vi "DAQmx.Dark.Current.SubVI.GenerateBooleanArray.vi"(8 "Activate: 1\nDeactivate: 0":bool, 11 "Tube":u8) -> (3 "Boolean array":bool[](array[boolean]))   [LabVIEW 2020]
panel:
  # "___"
  # "___"
  # "___"
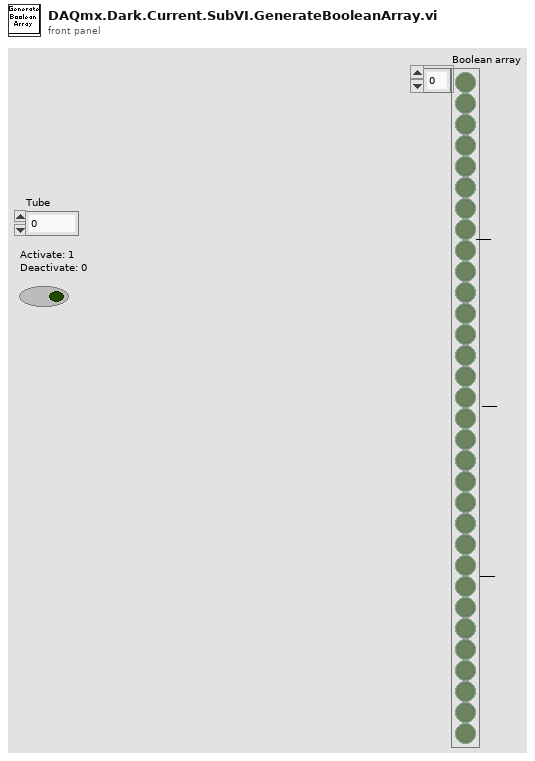
[diagram p1: front panel]
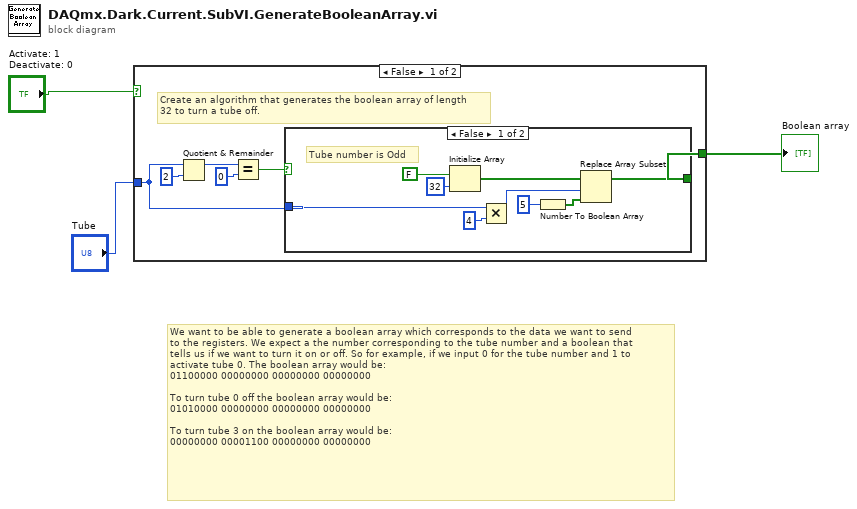
[diagram p0: block diagram]
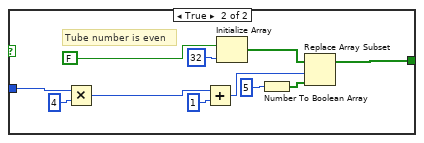
[diagram p2: hidden frame]
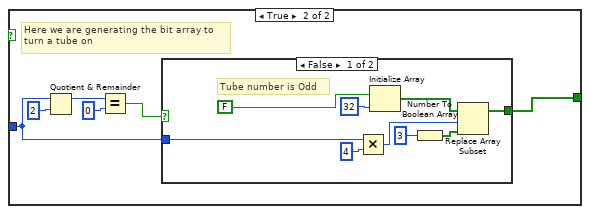
[diagram p3: hidden frame]
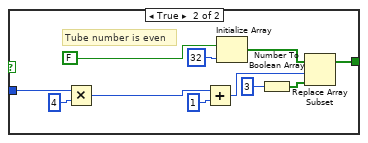
[diagram p4: hidden frame]
diagram:
  # "We want to be able to generate a boolean array which corresponds to the data we want to send \nto the registers. We expect a the number corresponding to the tube number and a boolean that\ntells us if we want to turn it on or off. So for example, if we input 0 for the tube number and 1 to\nactivate tube 0. The boolean array would be:\n01100000 00000000 00000000 00000000 \n\nTo turn tube 0 off the boolean array would be:\n01010000 00000000 00000000 00000000\n\nTo turn tube 3 on the boolean array would be:\n00000000 00001100 00000000 00000000"
  n1 = case shown="False" "Activate: 1\nDeactivate: 0" {
    tunnel: "Tube" -> [w5 w34]
    tunnel: [w6 w35] -> w1
    frame False {
      # "Create an algorithm that generates the boolean array of length\n32 to turn a tube off."
      n2 = Quotient & Remainder(x=w5, y=2) -> (x-y*floor(x/y)=w8:i32)  [unwired: 1 out]
      n3 = Equal?(x=w8, y=0) -> (x = y?=w4:bool)
      n4 = case shown="False" w4 {
        tunnel: w5 -> [w16 w24]
        tunnel: [w10 w25] -> w6
        frame False {
          # "Tube number is Odd"
          n5 = Initialize Array(FALSE, 32) -> (w12:bool[])
          n6 = Multiply(x=w16, y=4) -> (x*y=w11:i32)
          n7 = Number To Boolean Array(number=5) -> (Boolean array=w15:bool[])
          n8 = Replace Array Subset(array=w12, new element=w15, index=w11) -> (w10:bool[])
        }
        frame True {
          # "Tube number is even"
          n9 = Multiply(x=w24, y=4) -> (x*y=w20:i32)
          n10 = Add(x=w20, y=1) -> (x+y=w21:i32)
          n11 = Initialize Array(FALSE, 32) -> (w27:bool[])
          n12 = Number To Boolean Array(number=5) -> (Boolean array=w22:bool[])
          n13 = Replace Array Subset(array=w27, new element=w22, index=w21) -> (w25:bool[])
        }
      }
    }
    frame True {
      # "Here we are generating the bit array to \nturn a tube on"
      n14 = Quotient & Remainder(x=w34, y=2) -> (x-y*floor(x/y)=w32:i32)  [unwired: 1 out]
      n15 = Equal?(x=w32, y=0) -> (x = y?=w30:bool)
      n16 = case shown="False" w30 {
        tunnel: w34 -> [w39 w50]
        tunnel: [w37 w51] -> w35
        frame False {
          # "Tube number is Odd"
          n17 = Multiply(x=w39, y=4) -> (x*y=w38:i32)
          n18 = Initialize Array(FALSE, 32) -> (w42:bool[])
          n19 = Number To Boolean Array(number=3) -> (Boolean array=w36:bool[])
          n20 = Replace Array Subset(array=w42, new element=w36, index=w38) -> (w37:bool[])
        }
        frame True {
          # "Tube number is even"
          n21 = Multiply(x=w50, y=4) -> (x*y=w46:i32)
          n22 = Add(x=w46, y=1) -> (x+y=w47:i32)
          n23 = Initialize Array(FALSE, 32) -> (w53:bool[])
          n24 = Number To Boolean Array(number=3) -> (Boolean array=w48:bool[])
          n25 = Replace Array Subset(array=w53, new element=w48, index=w47) -> (w51:bool[])
        }
      }
    }
  }
  "Boolean array" <- w1
